vi "Modal Analysis of a Plate.vi"() -> ()   [LabVIEW 2023]
doc: "This example shows the application of the Time Series Analysis VIs in operational modal analysis.\n\nModal analysis is an experimental method that studies dynamic characteristics of a mechanical structure. Understanding the dynamic behavior of structures and structural components is becoming an increasingly important part of the design process for any mechanical system. Modal analysis can be implemented with either frequency-domain or time-domain methods.\n\nThis example obtains modal parameters (natural frequency, damping factor, modal shape) of an aluminum plate with a time-domain analysis method.\n\nA hammer impacts the aluminum plate and eight acceleration sensors located in different positions on the plate acquire the resulting vibration signals. Modal analysis is performed by completing the following steps:\n\n1) Build models for the multivariate time series in the time domain with the Prony method. The Prony method also is named the complex exponential method in the field of modal testing.\n2) Try different numbers of modes to form a mode histogram. In the mode histogram, frequency components of true modes do not change with different numbers of modes being computed. \n3) Select the true modes and compute the modal parameters again to obtain the natural frequency, damping ratio, and modal shape for each mode of the aluminum plate.\n\nYou can select <B>Mode Index</B> to see the corresponding modal shape, which indicates how the plate vibrates at a certain frequency.\n\nThis example uses the TSA Modal Parametric Modeling VI to estimate the modal parameters.\n\n<b>Instructions:</b>\n1) Run this VI.\n2) Change the mode index to see the animation of each modal shape."
uses:
  <vilib>/Native 3D Graph/xcontrol/3DPC_SurfacePlot.xctl
  <vilib>/addons/Time Series Analysis/Utilities.llb/TSA Data.ctl
  <vilib>/addons/Time Series Analysis/Modeling and Prediction.llb/TSA Vector Modal Parametric Modeling (Waveform).vi
  <vilib>/addons/_Advanced Signal Processing/NI_AdvSigProcTSA.lvlib
  <vilib>/Native 3D Graph/classes/Base Datatype.lvclass
panel:
  out "Vibration Signals of the Plate":waveform(dbl)[](graph)
  in  "Mode index (0-2)":i32 min=0 max=20 step=1
  out "Model Shape":refnum<class "Base Datatype.lvclass">[](xcontrol)
  in  "stop":bool
  in  "Number of modes":i32=16 min=2 max=1000 step=2
  out "Damping factors":dbl[](array[numeric])
  out "Frequencies (Hz)":dbl[](array[numeric])
  out "Mode Histogram":cluster{cluster{dbl, dbl}[]}[](graph)
  in  "Bin size (Hz)":dbl=2.0
  # "Overview: Shows the application of the Time Series Analysis VIs in operational modal analysis.\nRequirements: LabVIEW Full Development System, Advanced Signal Processing Toolkit\nInstructions: \n1. Run this VI.\n2. Change the mode index to see the animation of each modal shape.\n3. Click Stop to stop the VI."
  # "Modal Shape Animation"
  # "Modal Analysis"
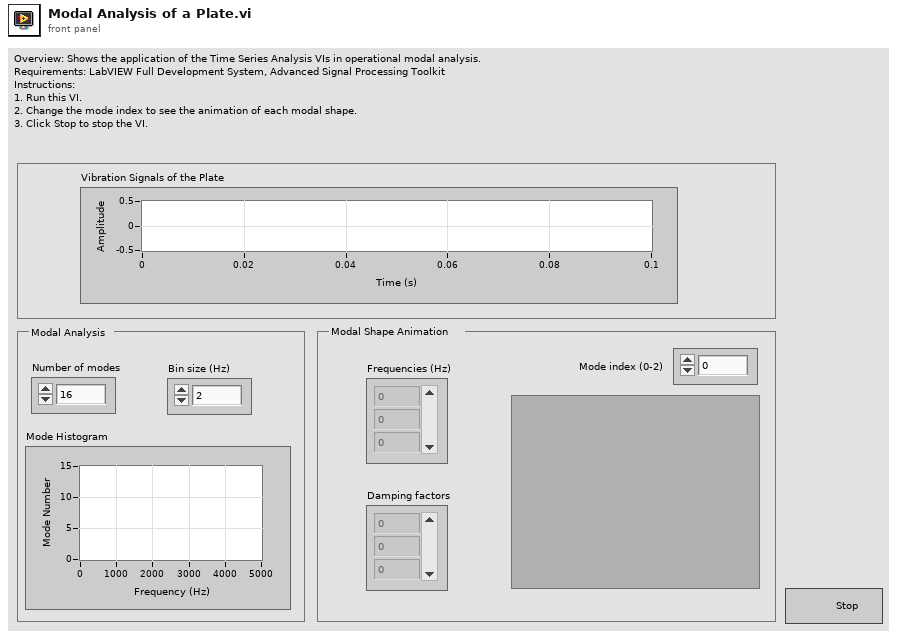
[diagram p1: front panel]
types:
  T1 = cluster{"frequency":dbl, "damping factor":dbl, "magnitude":dbl[], "phase":dbl[]}[]
  T2 = typedef "NI_AdvSigProcTSA.lvlib/TSA Data.ctl" = u16
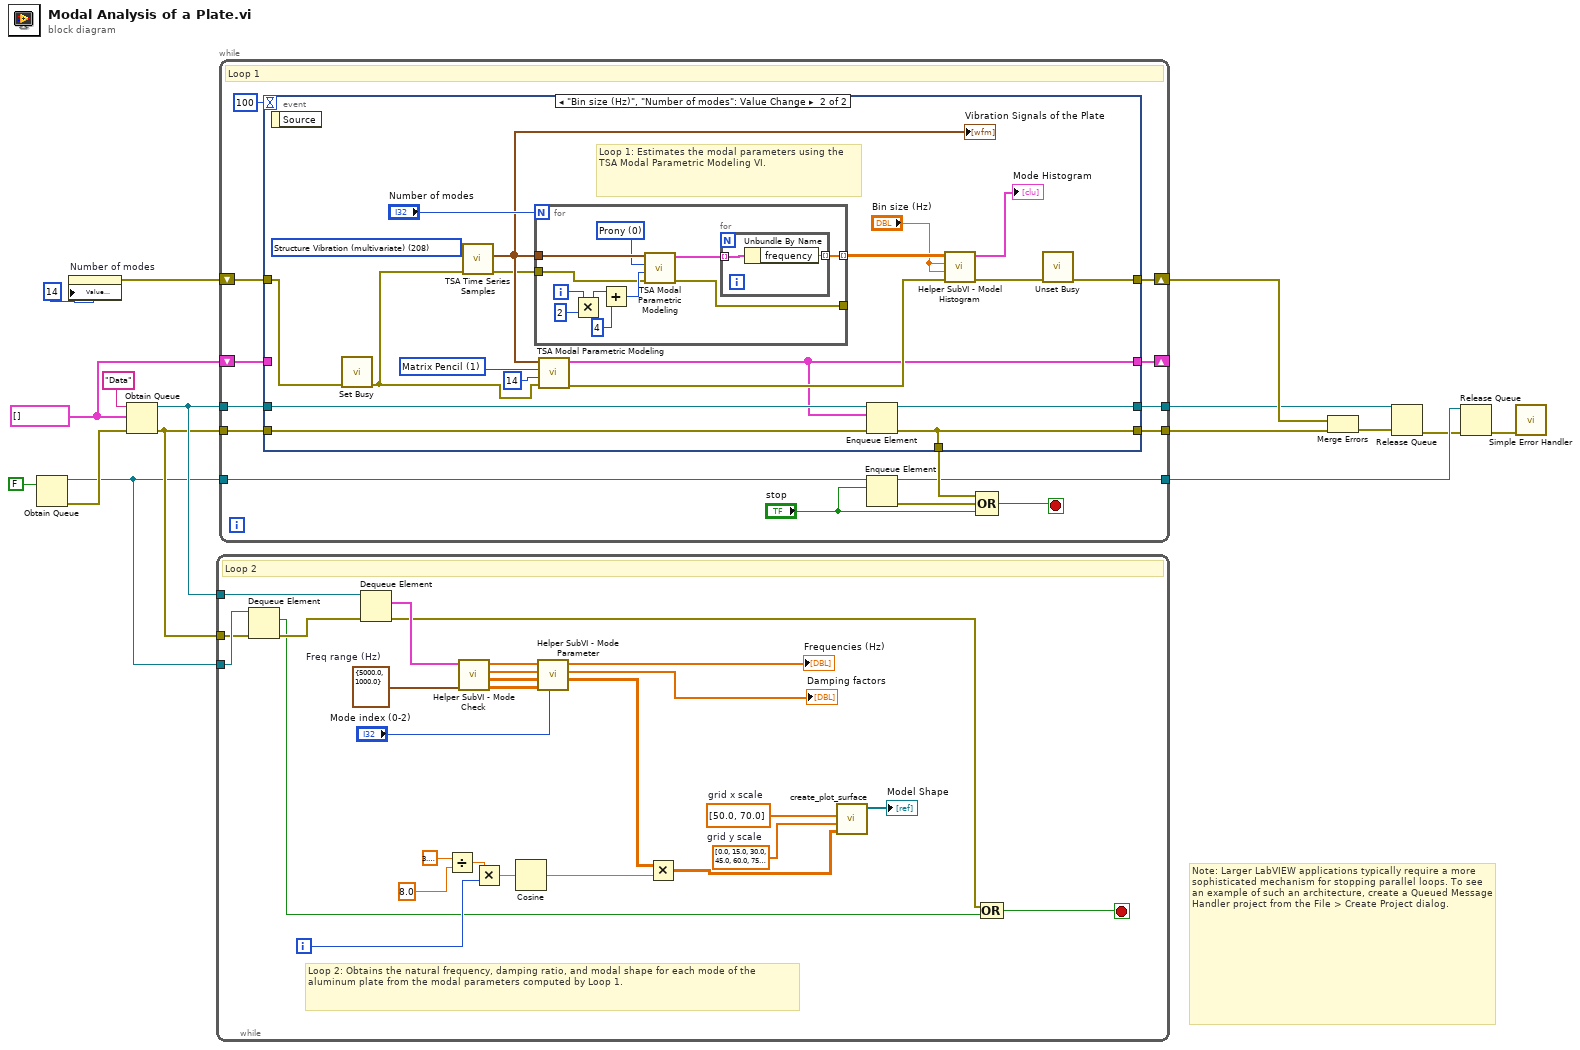
[diagram p0: block diagram]
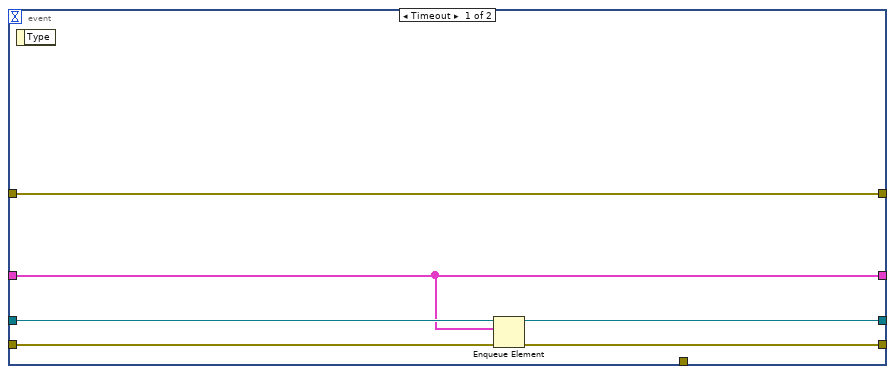
[diagram p2: hidden frame]
diagram:
  w12 = T1 [] ("frequency components")
  # "Note: Larger LabVIEW applications typically require a more sophisticated mechanism for stopping parallel loops. To see an example of such an architecture, create a Queued Message Handler project from the File > Create Project dialog."
  n1 = Obtain Queue(element data type=FALSE) -> (queue out=w6:refnum<queue>, error out=w7:errorcluster)  [unwired: 4 in, 1 out]
  n2 = property on="Number of modes" class="DigNum (strict)"("Value (Signaling)"=14) -> (error out=w11:errorcluster)  [unwired: 2 in, 1 out]
  n3 = Obtain Queue(name (unnamed)="Data", element data type=w12, error in (no error)=w7) -> (queue out=w14:refnum<queue>, error out=w13:errorcluster)  [unwired: 2 in, 1 out]
  n4 = while {
    tunnel: w14 -> [w28]
    tunnel: w13 -> [w25]
    tunnel: w6 -> [w26]
    i -> [w43]
    stop <- w21 stop-if-true
    w34 = cluster{"high":dbl, "low":dbl} {"high"=5000.0, "low"=1000.0}  # Freq range (Hz)
    w19 = dbl[] [0.0, 15.0, 30.0, 45.0, 60.0, 75.0, 90.0]  # grid y scale
    w20 = dbl[] [50.0, 70.0]  # grid x scale
    # "Loop 2: Obtains the natural frequency, damping ratio, and modal shape for each mode of the aluminum plate from the modal parameters computed by Loop 1."
    # "Loop 2"
    n5 = Dequeue Element(queue=w26, error in (no error)=w25) -> (element=w22:bool, error out=w24:errorcluster)  [unwired: 1 in, 2 out]
    n6 = Dequeue Element(queue=w28, error in (no error)=w24) -> (element=w27:T1, error out=w23:errorcluster)  [unwired: 1 in, 2 out]
    n7 = Divide(x=3.141592653589793 ("Pi"), y=8.0) -> (x/y=w38:dbl)
    n8 = call "Helper SubVI - Mode Check.vi"("freq range"=w34, "frequency components"=w27) -> ("phase"=w35:dbl[][], "mag"=w33:dbl[][], "damping factor"=w32:dbl[], "freq"=w31:dbl[])  [unwired: 6 in]
    n9 = Multiply(x=w38, y=w43) -> (x*y=w40:dbl)
    n10 = Cosine(x=w40) -> (cos(x)=w39:dbl)
    n11 = call "Helper SubVI - Mode Parameter.vi"("mode index"="Mode index (0-2)", "phase"=w35, "mag"=w33, "damping in"=w32, "freq in"=w31) -> ("mode shape"=w36:dbl[][], "damping out"=→"Damping factors":dbl[], "freq out"=→"Frequencies (Hz)":dbl[])  [unwired: 3 in, 1 out]
    n12 = Multiply(x=w36, y=w39) -> (x*y=w18:dbl[][])
    n13 = call <vilib>:"create_plot_surface.vi"("z matrix"=w18, "y vector"=w19, "x vector"=w20) -> ("plots out"=→"Model Shape":refnum<class "Base Datatype.lvclass">[])  [unwired: 2 in, 6 out]
    n14 = Compound Arithmetic op=OR(w23, w22) -> (w21:bool)
  }
  n15 = while {
    shift-right: [w57] -> w10
    shift-left: w11 -> [w56]
    shift-right: [w51] -> _
    shift-left: w12 -> [w50]
    tunnel: w14 -> [w55]
    tunnel: [w53] -> w4
    tunnel: w13 -> [w54]
    tunnel: [w52] -> w5
    tunnel: w6 -> [w47]
    tunnel: [w45] -> w3
    stop <- w48 stop-if-true
    # "Loop 1"
    n16 = event shown="[1] \"Bin size (Hz)\", \"Number of modes\": Value Change" {
      selector: _ -> [_ _]
      dyn-events: _ -> [_ _]
      timeout: 100 -> [_ _]
      tunnel: [w64 w71] -> w57
      tunnel: w56 -> [w64 w70]
      tunnel: w55 -> [w63 w69]
      tunnel: w54 -> [w62 w68]
      tunnel: [w60 w67] -> w53
      tunnel: [w59 w65] -> w52
      tunnel: [w61 w66] -> w51
      tunnel: w50 -> [w61 _]
      tunnel: [_ w65] -> w49
      event Timeout {
        n17 = event-data() -> ()  [unwired: 2 out]
        n18 = Enqueue Element(queue=w63, element=w61, error in (no error)=w62) -> (queue out=w60:refnum<queue>, error out=w59:errorcluster)  [unwired: 2 out]
      }
      event "Bin size (Hz)", "Number of modes": Value Change {
        w75 = T2 208 items=["Kobe Earthquake"=201, "EEG"=210, "Bearing Vibration (simulated)"=211, "Period Product Sales"=214, "Beam Vibration (nonlinear)"=217, "Beam Vibration (linear)"=218, "Signal With Echo"=219, "Engine Knocking"=220, "Power Line"=221, "-"=200, "Beam Deflections (multivariate)"=207, "Structure Vibration (multivariate)"=208, "Human MEG (multivariate)"=222] ("data")
        w79 = u16 1 items=["Prony", "Matrix Pencil"] ("method")
        # "Loop 1: Estimates the modal parameters using the TSA Modal Parametric Modeling VI."
        n19 = event-data() -> ()  [unwired: 2 out]
        n20 = call <vilib>:"Set Busy.vi"("error in (no error)"=w70) -> ("error out"=w74:errorcluster)  [unwired: 3 in, 7 out]
        n21 = call <vilib>:"TSA Time Series Samples.vi"("error in (no error)"=w74, "data"=w75) -> ("error out"=w73:errorcluster, "multivariate time series"=w77:waveform(dbl)[])  [unwired: 8 out]
        "Vibration Signals of the Plate" <- w77
        n22 = for {
          N: "Number of modes" -> [_]
          tunnel: [w86] -> w81 mode=indexing
          tunnel: w77 -> [w93]
          tunnel: [w85] -> _
          tunnel: w73 -> [w84]
          i -> [w89]
          w87 = u16 0 items=["Prony", "Matrix Pencil"] ("method")
          n23 = Multiply(x=w89, y=2) -> (x*y=w88:i32)
          n24 = Add(x=w88, y=4 ("x")) -> (x+y=w91:i32)
          n25 = call-poly <vilib>:"TSA Modal Parametric Modeling.vi"("error in (no error)"=w84, "model order"=w91, "method"=w87, "Xt"=w93) -> ("error out"=w85:errorcluster, "frequency components"=w94:T1)  [unwired: 6 out]
          n26 = for {
            tunnel: w94 -> [w96] mode=indexing
            tunnel: [w95] -> w86 mode=indexing
            n27 = Unbundle By Name(w96) -> ("frequency"=w95:dbl)
          }
        }
        n28 = call-poly <vilib>:"TSA Modal Parametric Modeling.vi"("error in (no error)"=w74, "model order"=14 ("num of components"), "method"=w79, "Xt"=w77) -> ("error out"=w72:errorcluster, "frequency components"=w66:T1)  [unwired: 6 out]
        n29 = Enqueue Element(queue=w69, element=w66, error in (no error)=w68) -> (queue out=w67:refnum<queue>, error out=w65:errorcluster)  [unwired: 2 out]
        n30 = call "Helper SubVI - Model Histogram.vi"("error in (no error)"=w72, "step size (Hz)"="Bin size (Hz)", "range (Hz)"="Bin size (Hz)", "freq (Hz)"=w81) -> ("error out"=w78:errorcluster, "Mode Histogram"=→"Mode Histogram":cluster{cluster{dbl, dbl}[]}[])  [unwired: 6 out]
        n31 = call <vilib>:"Unset Busy.vi"("error in (no error)"=w78) -> ("error out"=w71:errorcluster)  [unwired: 1 in, 9 out]
      }
    }
    n32 = Enqueue Element(queue=w47, element="stop") -> (queue out=w45:refnum<queue>, error out=w44:errorcluster)  [unwired: 1 in, 2 out]
    n33 = Compound Arithmetic op=OR(w49, w44, "stop") -> (w48:bool)
  }
  n34 = Merge Errors(w10, w5) -> (w9:errorcluster)
  n35 = Release Queue(queue=w4, error in (no error)=w9) -> (error out=w2:errorcluster)  [unwired: 1 in, 2 out]
  n36 = Release Queue(queue=w3, error in (no error)=w2) -> (error out=w1:errorcluster)  [unwired: 1 in, 2 out]
  n37 = call <vilib>:"Simple Error Handler.vi"("error in (no error)"=w1) -> ()  [unwired: 4 in, 5 out]
